vi "Copy Data.vi"(0 "AOAIRefs":T2[](array[typedef]), 5 "Old type":T1, 9 "New type":T1, 11 "error in (no error)":errorcluster) -> (15 "error out":errorcluster)   [LabVIEW 2020, in "PXISlotGP.xctl"]
uses:
  PXISlotGP.xctl
  AOAIRefs.ctl
  PXISlot XControl/Connector Type.ctl
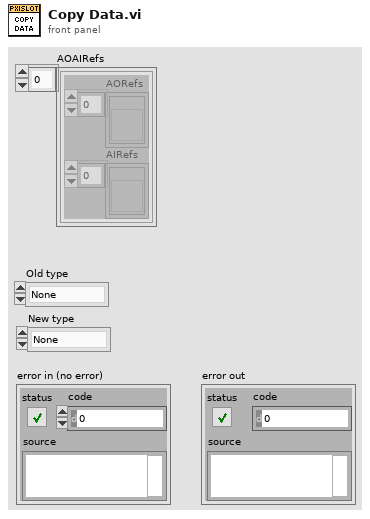
[diagram p1: front panel]
types:
  T1 = typedef "Connector Type.ctl" = enum16{"None", "PXI-4461", "BNC-2110", "BNC-2090", "PXIe-4463", "PXIe-4464"}
  T2 = typedef "AOAIRefs.ctl" = cluster{"AORefs":refnum<vi>[], "AIRefs":refnum<vi>[]}
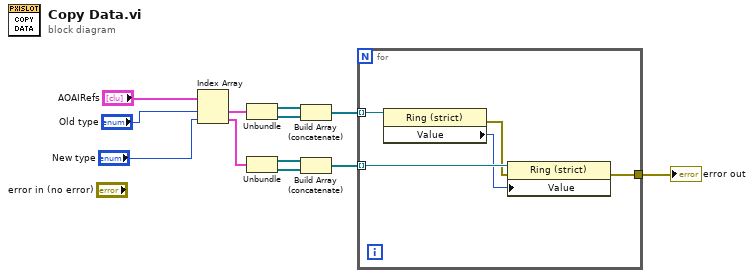
[diagram p0: block diagram]
diagram:
  n1 = Index Array(array="AOAIRefs", index #1="Old type", index #2="New type") -> (element #1=w10:T2, element #2=w5:T2)
  n2 = Unbundle(w10) -> ("AORefs"=w9:refnum<vi>[], "AIRefs"=w8:refnum<vi>[])
  n3 = Unbundle(w5) -> ("AORefs"=w7:refnum<vi>[], "AIRefs"=w6:refnum<vi>[])
  n4 = Build Array (concatenate)(w9, w8) -> (w4:refnum<vi>[])
  n5 = Build Array (concatenate)(w7, w6) -> (w3:refnum<vi>[])
  n6 = for {
    tunnel: w4 -> [w17] mode=indexing
    tunnel: w3 -> [w16] mode=indexing
    tunnel: [w13] -> w2
    n7 = property class="Ring (strict)"(reference=w17) -> (error out=w14:errorcluster, "Value"=w15:u16)  [unwired: 1 in, 1 out]
    n8 = property class="Ring (strict)"(reference=w16, error in=w14, "Value"=w15) -> (error out=w13:errorcluster)  [unwired: 1 out]
  }
  "error out" <- w2
